vi "Copy Class.vi"(10 "Template Path":path, 11 "Second Library Script Strategy in":refnum<class "Second Library Script Strategy.lvclass">) -> (0 "error out":errorcluster, 3 "Second Library Script Strategy out":refnum<class "Second Library Script Strategy.lvclass">)   [LabVIEW 2021, in "_Create From Template.lvlib" / "Script Strategy.lvlib" / "Second Library Script Strategy.lvclass"]
uses:
  Second Library Script Strategy.lvclass
  Second Library Script Strategy.lvclass/Second Library Script Strategy.ctl
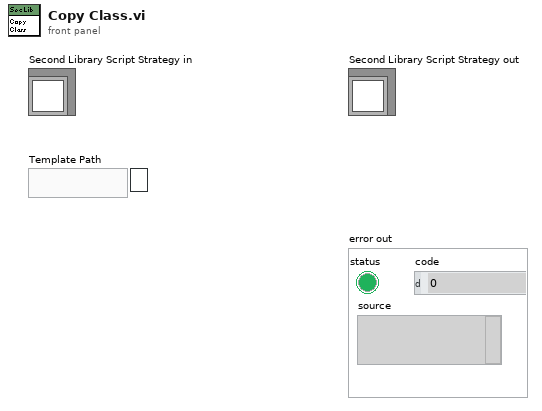
[diagram p1: front panel]
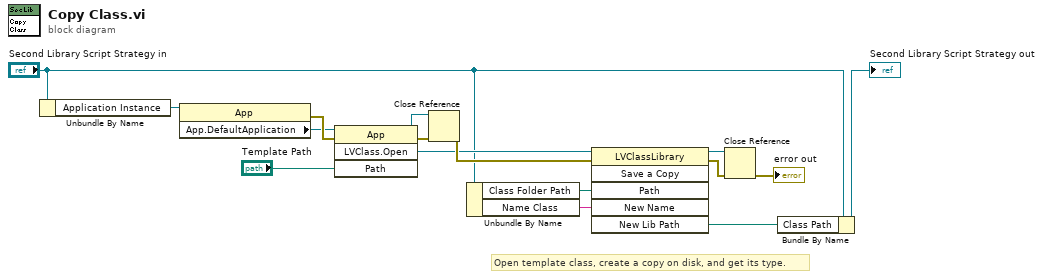
[diagram p0: block diagram]
diagram:
  # "Open template class, create a copy on disk, and get its type."
  n1 = Unbundle By Name("Second Library Script Strategy in") -> ("Application Instance"=w7:refnum<vi>)
  n2 = property class="App"(reference=w7) -> (error out=w15:errorcluster, "App.DefaultApplication"=w9:refnum<vi>)  [unwired: 1 in, 1 out]
  n3 = invoke class="App" method="LVClass.Open"(reference=w9, error in=w15, "Path"="Template Path") -> (reference out=w8:refnum<vi>, error out=w16:errorcluster, "LVClass.Open"=w11:refnum<vi>)  [unwired: 1 in, 1 out]
  n4 = Close Reference(reference=w8, error in (no error)=w16) -> (error out=w13:errorcluster)
  n5 = Unbundle By Name("Second Library Script Strategy in") -> ("Class Folder Path"=w5:path, "Name Class"=w6:string)
  n6 = invoke class="LVClassLibrary" method="Save a Copy"(reference=w11, error in=w13, "Path"=w5, "New Name"=w6) -> (reference out=w10:refnum<vi>, error out=w1:errorcluster, "New Lib Path"=w2:path)  [unwired: 2 in, 3 out]
  n7 = Close Reference(reference=w10, error in (no error)=w1) -> (error out=→"error out":errorcluster)
  n8 = Bundle By Name(cluster="Second Library Script Strategy in", "Class Path"=w2) -> (→"Second Library Script Strategy out":refnum<class "Second Library Script Strategy.lvclass">)
